vi "CAN Semaphore Ref FGV.vi"(6 "CAN FGV State":T2=enum."Get", 8 "error in":errorcluster, 10 "Current Scoket":i16, 11 "semaphore In":T1) -> (0 "error out":errorcluster, 3 "Semaphore Out":T1[](array[typedef]))   [LabVIEW 2023, in "LTT_TeststandSteptypes.lvlib"]
uses:
  LTT_TeststandSteptypes.lvlib
  Control/CAN FGV State.ctl
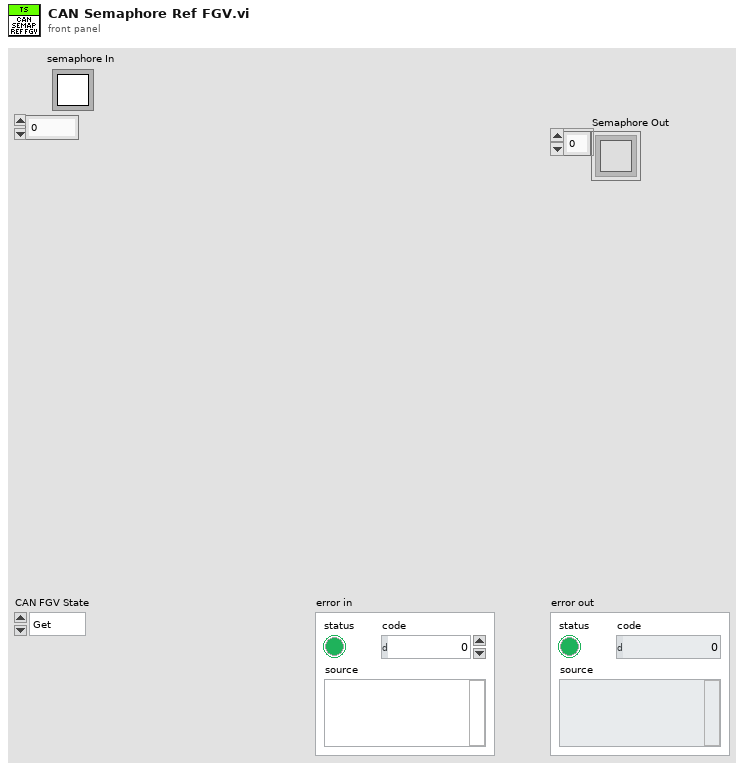
[diagram p1: front panel]
types:
  T1 = typedef "Semaphore RefNum" = refnum<k1>
  T2 = typedef "LTT_TeststandSteptypes.lvlib/CAN FGV State.ctl" = enum16{"Init", "Get", "Set"}
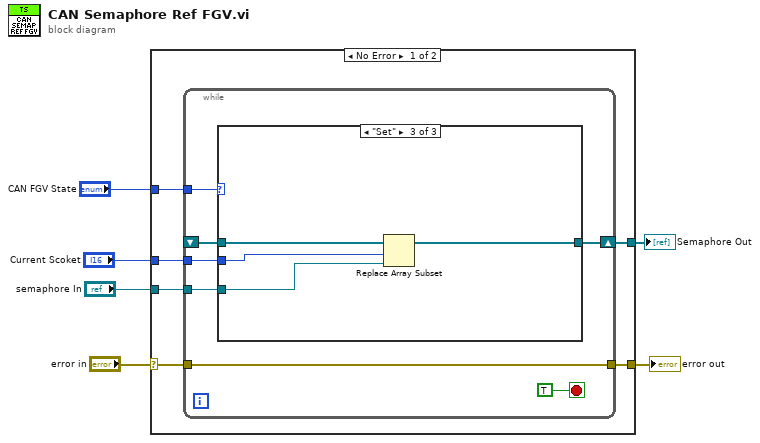
[diagram p0: block diagram]
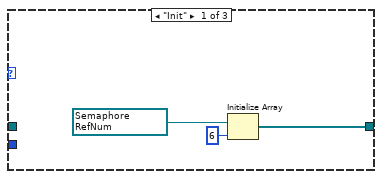
[diagram p2: hidden frame]
diagram:
  n1 = case shown="No Error" "error in" {
    selector: "error in" -> [w12 w28]
    tunnel: "CAN FGV State" -> [w11 _]
    tunnel: [w10 w28] -> w4
    tunnel: [w9 _] -> w1
    tunnel: "semaphore In" -> [w8 _]
    tunnel: "Current Scoket" -> [w7 _]
    frame No Error {
      n2 = while {
        tunnel: w12 -> [w15]
        tunnel: w11 -> [w18]
        shift-right: [w17] -> w9
        shift-left: _ -> [w16]
        tunnel: [w15] -> w10
        tunnel: w8 -> [w14]
        tunnel: w7 -> [w13]
        stop <- TRUE stop-if-true
        n3 = case shown="\"Set\"" w18 {
          tunnel: [w20 w23 w26] -> w17
          tunnel: w16 -> [_ w23 w27]
          tunnel: w14 -> [_ _ w25]
          tunnel: w13 -> [_ _ w24]
          frame "Init" {
            w22 = T1 refnum items=["semaphore"] ("semaphore")
            n4 = Initialize Array(w22, 6 ("dimension size")) -> (w20:T1[])
          }
          frame "Get", Default {
          }
          frame "Set" {
            n5 = Replace Array Subset(array=w27, new element=w25, index=w24) -> (w26:T1[])
          }
        }
      }
    }
    frame Error {
    }
  }
  "error out" <- w4
  "Semaphore Out" <- w1
